vi "Byte To SPOS.vi"(11 "Numeric":u8) -> (3 "SPOS":T1)   [LabVIEW 2022 SP3, in "FHPP.lvclass"]
uses:
  FHPP.lvclass
  FHPP.lvclass/FHPP.ctl
  TypeDefs/SPOS.ctl
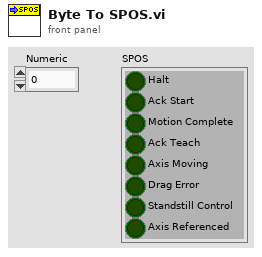
[diagram p1: front panel]
types:
  T1 = typedef "FHPP.lvclass/SPOS.ctl" = cluster{"Halt":bool, "Ack Start":bool, "Motion Complete":bool, "Ack Teach":bool, "Axis Moving":bool, "Drag Error":bool, "Standstill Control":bool, "Axis Referenced":bool}
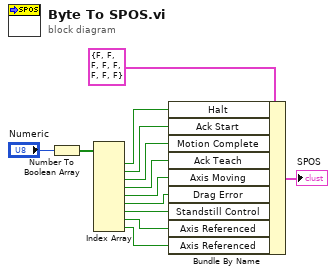
[diagram p0: block diagram]
diagram:
  n1 = Number To Boolean Array(number="Numeric") -> (Boolean array=w4:bool[])
  n2 = Index Array(array=w4) -> (element #1=w5:bool, element #2=w6:bool, element #3=w7:bool, element #4=w8:bool, element #5=w9:bool, element #6=w10:bool, element #7=w11:bool, element #8=w12:bool, element #9=w13:bool)  [unwired: 9 in]
  n3 = Bundle By Name(cluster=T1 {"Halt"=FALSE, "Ack Start"=FALSE, "Motion Complete"=FALSE, "Ack Teach"=FALSE, "Axis Moving"=FALSE, "Drag Error"=FALSE, "Standstill Control"=FALSE, "Axis Referenced"=FALSE} ("SPOS"), "Halt"=w5, "Ack Start"=w6, "Motion Complete"=w7, "Ack Teach"=w8, "Axis Moving"=w9, "Drag Error"=w10, "Standstill Control"=w11, "Axis Referenced"=w12, "Axis Referenced"=w13) -> (→"SPOS":T1)
